vi "FindPositionParticle1.vi"(2 "X,Y (2Frame)":dbl[](array[numeric]), 3 "X,Y (1Frame)":dbl[](array[numeric]), 4 "Y2":dbl, 5 "X2":dbl, 6 "Y1":dbl, 7 "X1":dbl) -> (0 "Index X2":i32, 1 "Index X1":i32)   [LabVIEW 2017]
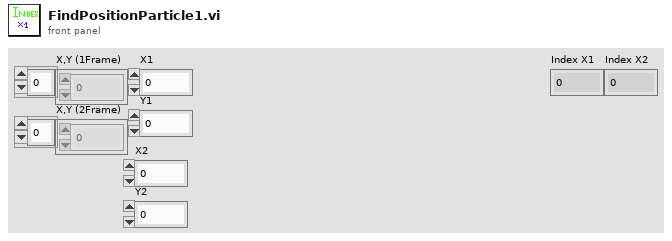
[diagram p1: front panel]
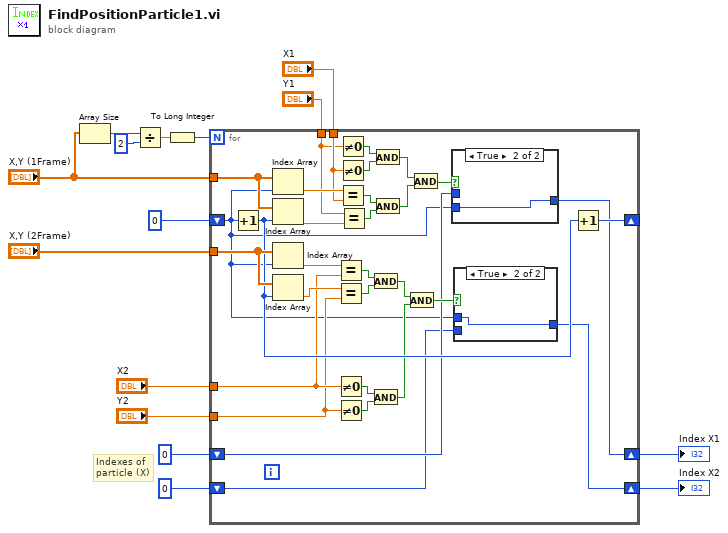
[diagram p0: block diagram]
diagram:
  # "Indexes of \nparticle (X)"
  n1 = Array Size(array="X,Y (1Frame)") -> (size(s)=w15:i32)
  n2 = Divide(x=w15, y=2) -> (x/y=w13:dbl)
  n3 = To Long Integer(number=w13) -> (32bit integer=w12:i32)
  n4 = for {
    N: w12 -> [_]
    tunnel: "X,Y (1Frame)" -> [w46]
    tunnel: "X,Y (2Frame)" -> [w45]
    shift-right: [w17] -> w1
    shift-left: 0 -> [w16]
    shift-right: [w19] -> w2
    shift-left: 0 -> [w20]
    shift-right: [w43] -> _
    shift-left: 0 -> [w18]
    tunnel: "X2" -> [w25]
    tunnel: "Y2" -> [w24]
    tunnel: "X1" -> [w40]
    tunnel: "Y1" -> [w39]
    n5 = Increment(x=w18) -> (x+1=w44:i32)
    n6 = Index Array(array=w46, index=w18) -> (element=w42:dbl)
    n7 = Index Array(array=w46, index=w44) -> (element=w41:dbl)
    n8 = Index Array(array=w45, index=w18) -> (element=w27:dbl)
    n9 = Index Array(array=w45, index=w44) -> (element=w26:dbl)
    n10 = Equal?(x=w27, y=w25) -> (x = y?=w29:bool)
    n11 = Equal?(x=w26, y=w24) -> (x = y?=w28:bool)
    n12 = Not Equal To 0?(x=w25) -> (x != 0?=w31:bool)
    n13 = Not Equal To 0?(x=w24) -> (x != 0?=w30:bool)
    n14 = Not Equal To 0?(x=w39) -> (x != 0?=w38:bool)
    n15 = Not Equal To 0?(x=w40) -> (x != 0?=w37:bool)
    n16 = Equal?(x=w42, y=w40) -> (x = y?=w36:bool)
    n17 = Equal?(x=w39, y=w41) -> (x = y?=w35:bool)
    n18 = And(x=w29, y=w28) -> (x .and. y?=w22:bool)
    n19 = And(x=w31, y=w30) -> (x .and. y?=w23:bool)
    n20 = And(x=w38, y=w37) -> (x .and. y?=w34:bool)
    n21 = And(x=w36, y=w35) -> (x .and. y?=w33:bool)
    n22 = And(x=w22, y=w23) -> (x .and. y?=w21:bool)
    n23 = And(x=w34, y=w33) -> (x .and. y?=w32:bool)
    n24 = case shown="True" w32 {
      tunnel: w20 -> [w49 _]
      tunnel: w18 -> [_ w50]
      tunnel: [w49 w50] -> w19
      frame False {
      }
      frame True {
      }
    }
    n25 = case shown="True" w21 {
      tunnel: w18 -> [_ w48]
      tunnel: [w47 w48] -> w17
      tunnel: w16 -> [w47 _]
      frame False {
      }
      frame True {
      }
    }
    n26 = Increment(x=w44) -> (x+1=w43:i32)
  }
  "Index X1" <- w2
  "Index X2" <- w1
